vi "Multi_moments_LDA+_An.vi"(3 "Timescales":dbl[](array[numeric]), 4 "Measurement top level?":bool, 6 "Vari Spaced":dbl[][](array[numeric]) format="%.2f") -> (1 "Channel Values":string[](array[string]))   [LabVIEW 2011]
uses:
  Controls/Post_Process.ctl
  Globals/Meas_global.vi
  Globals/Trav_pos_global.vi
  Globals/Dynamic_call_global.ph.vi
  Globals/LDA_meas_global_1.vi
  Acquisition/PWA/PWAtasksGLOBAL.vi
panel:
  out "Channel Names":string[](array[string])
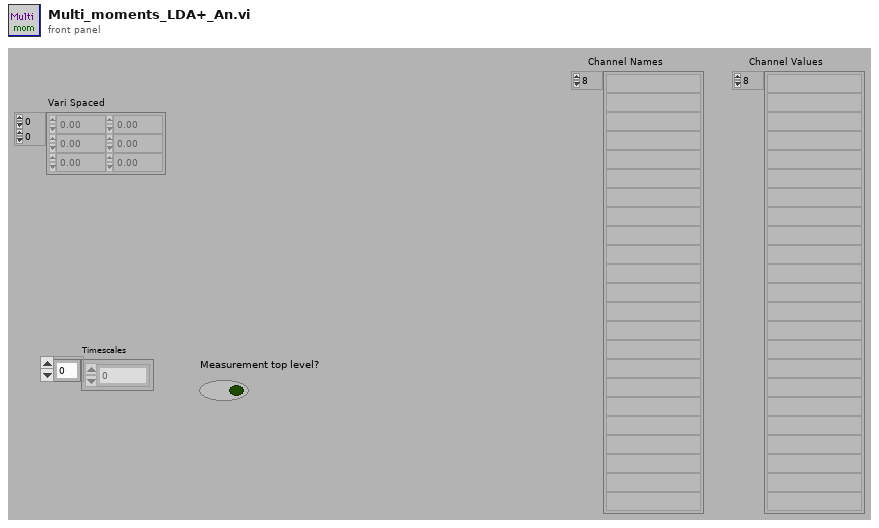
[diagram p1: front panel]
types:
  T1 = typedef "Analysis_info_cluster.ctl" = cluster{"Colour":u32, "Inst type":T2, "Inst name":string, "Symbol":string, "Code name":string, "Extra Info":string, "Inst Array":T3, "Index":i32, "Voltage Index":i32, "Extra Titles":string[], "Extra Values":string[], "Eng Values":dbl[], "Time (ms)":dbl[], "TT / Voltage":dbl[], "U":dbl, "u^2":dbl, "u^3":dbl, "u^4":dbl, "Skew_u":dbl, "Kurt_u":dbl, "Sd Error in Mean":dbl, "% u'/U":dbl, "X":dbl, "Y":dbl, "Z":dbl, "Spectra":T4, "Autocorrelation":T4, "Timescale integral to 25%":dbl, "Sd Error in Variance":dbl, "Calib File":path, "Calib Constants":dbl[], "Histogram":T4, "Output Position":bool, "Full Stats":bool}
  T2 = typedef "Inst_type.ctl" = enum16{"Propeller anemometer", "Raw voltage", "Pressure Transducer", "Pitot-static tube", "Preston tube", "Hot wire", "Cross wire 1", "Cross wire 2", "Generic Linear", "Generic Polynomial", "Generic BackPoly", "Fast FID", "Thermocouple", "Cold wire", "Pulsed Wire", "LDA Vel", "LDA Tran time", "LDA Arr time"}
  T3 = typedef "Instrument_Array.ctl" = enum16{"PWA", "LDA", "Analogue"}
  T4 = typedef "XY_Plot_Cluster.ctl" = cluster{"First Name":string, "Second Name":string, "X axis name":string, "Y axis name":string, "X array":dbl[], "Y array":dbl[]}
  T5 = typedef "Post_Process.ctl" = enum16{"Take New Data", "Post Process Raw Data File"}
  T6 = typedef "PWA_Data.ctl" = enum16{"No PWA Data", "One Ch PWA"}
  T7 = cluster{"Name":string, "X":dbl, "Y":dbl, "Z":dbl}[]
  T8 = typedef "Correlation_cluster1.ctl" = cluster{"U inst":string, "uw":dbl, "u^2w":dbl, "uw^2":dbl, "uw/u'w'":dbl, "W inst":string, "uw^3":dbl, "u^3w":dbl, "u^2w^2":dbl, "Index U":i32, "Index W":i32}
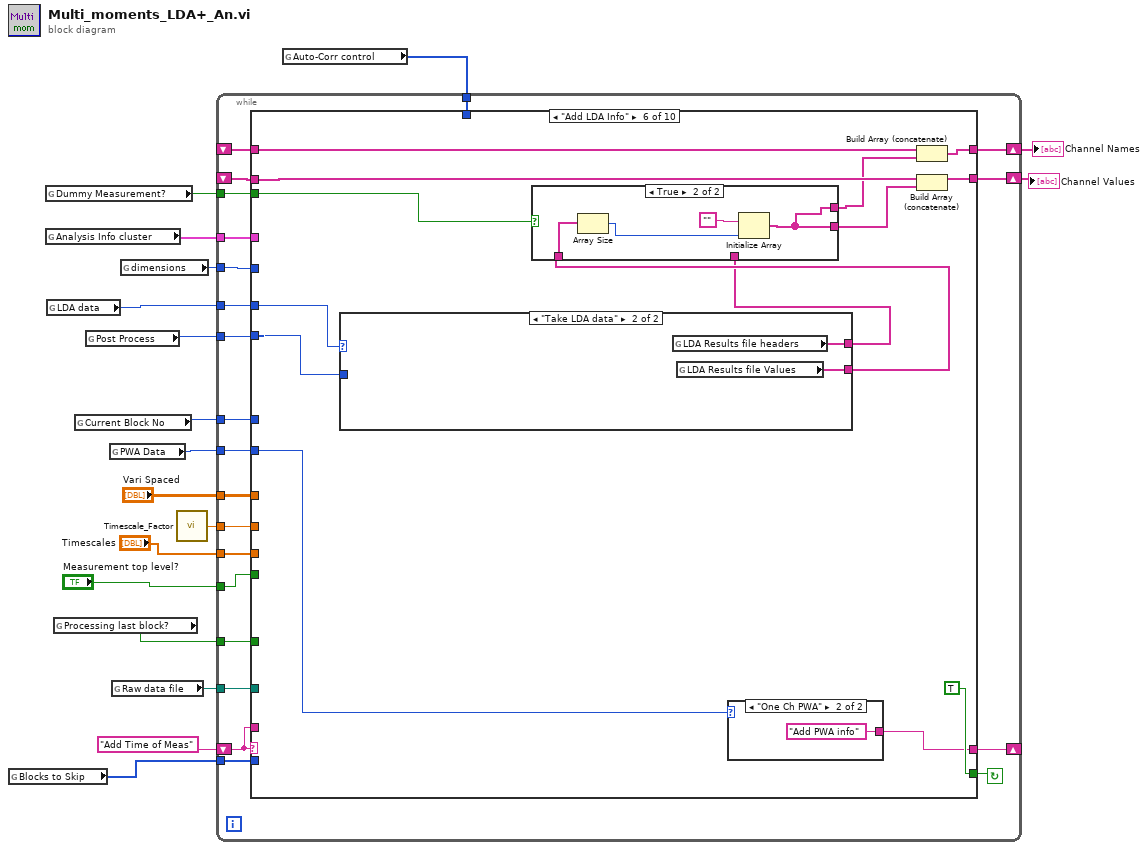
[diagram p0: block diagram]
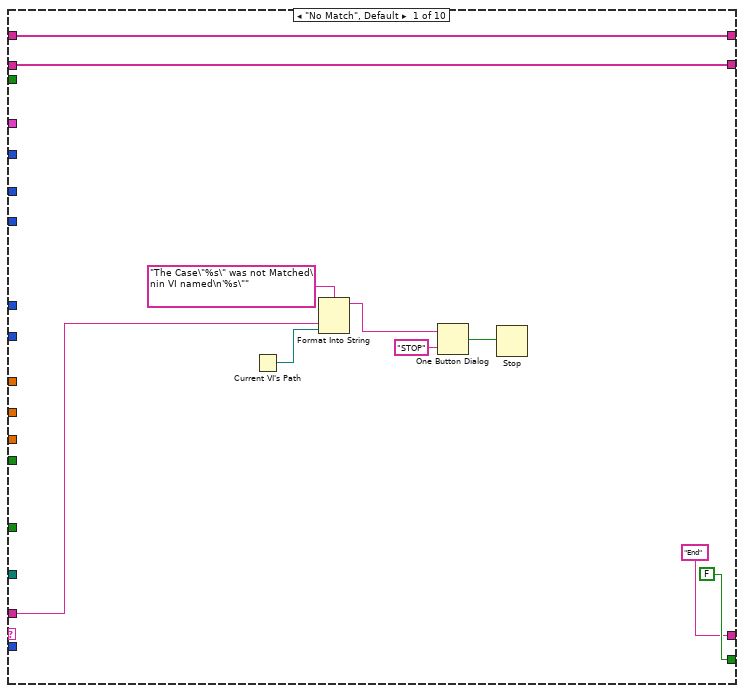
[diagram p2: hidden frame]
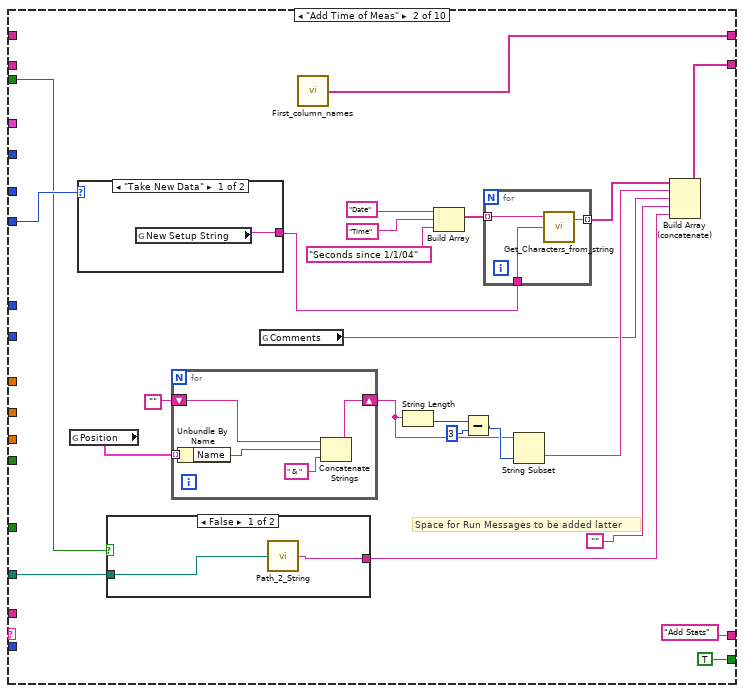
[diagram p3: hidden frame]
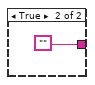
[diagram p4: hidden frame]
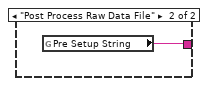
[diagram p5: hidden frame]
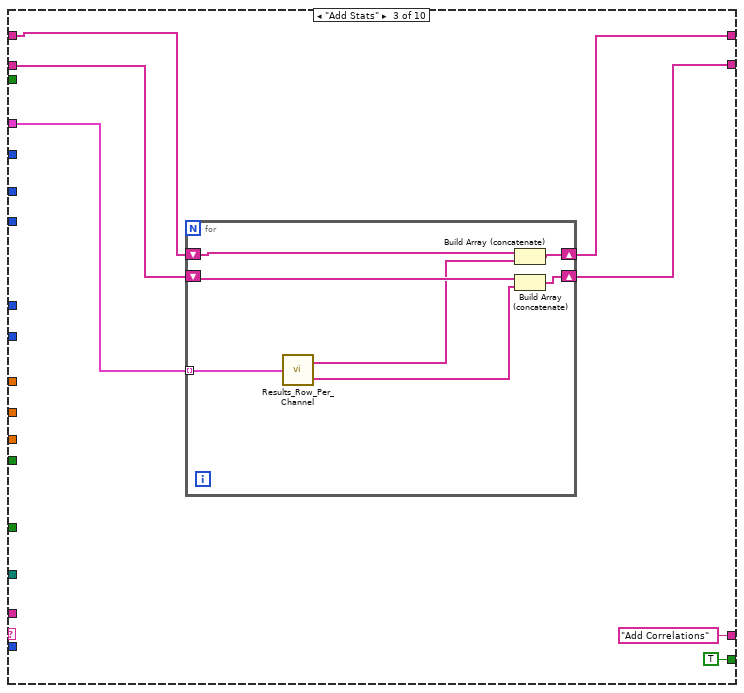
[diagram p6: hidden frame]
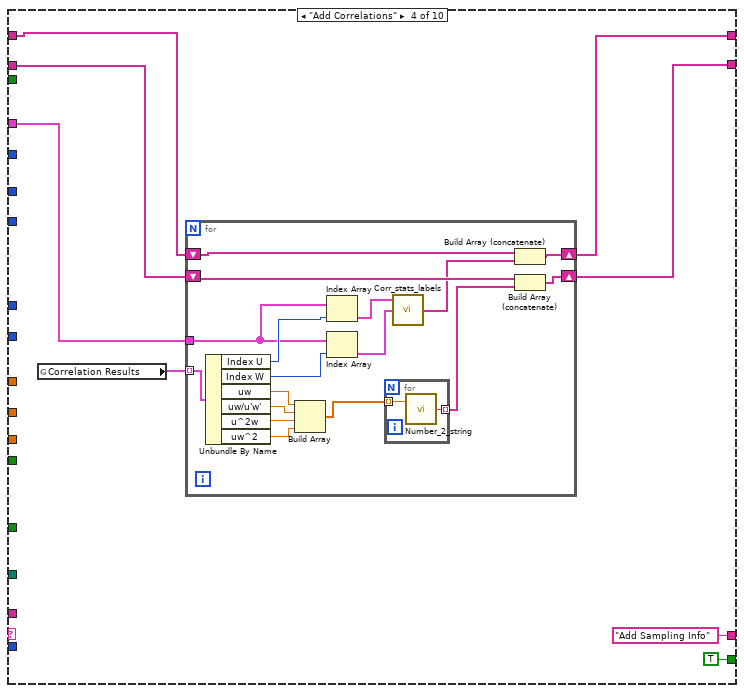
[diagram p7: hidden frame]
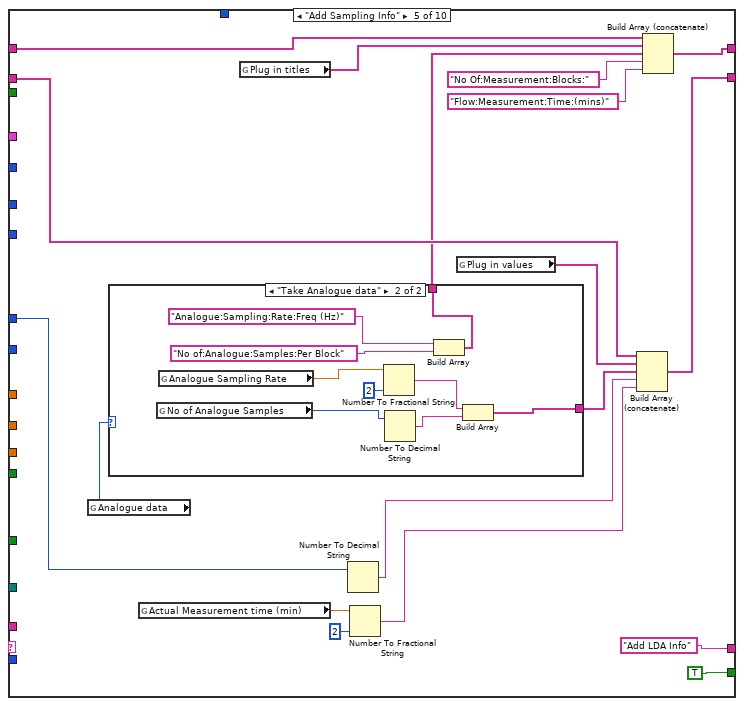
[diagram p8: hidden frame]
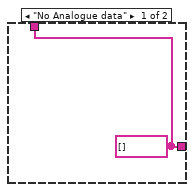
[diagram p9: hidden frame]
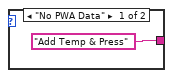
[diagram p10: hidden frame]
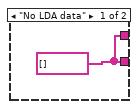
[diagram p12: hidden frame]
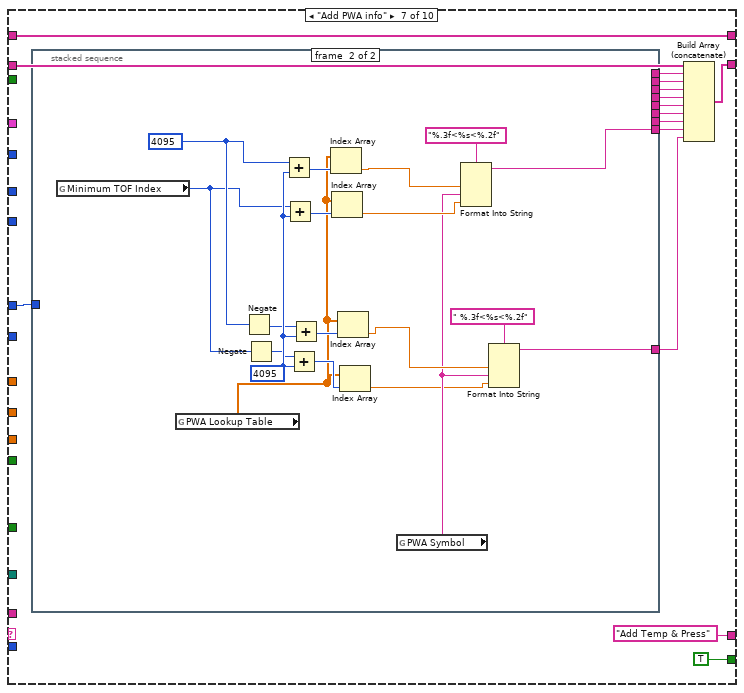
[diagram p13: hidden frame]
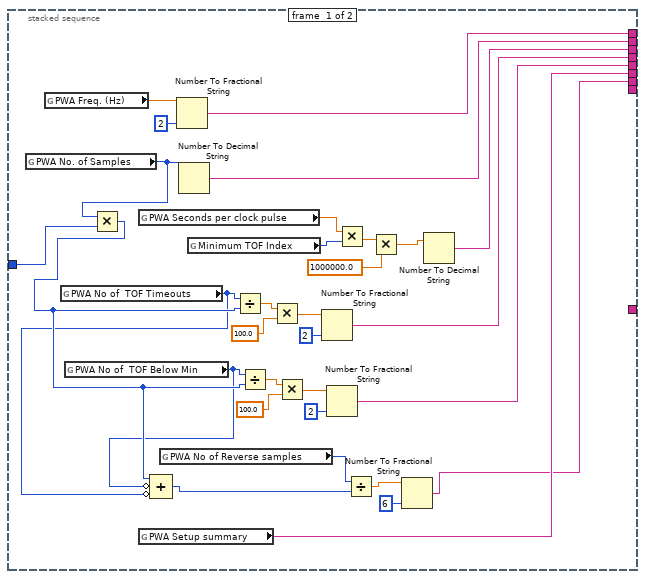
[diagram p14: hidden frame]
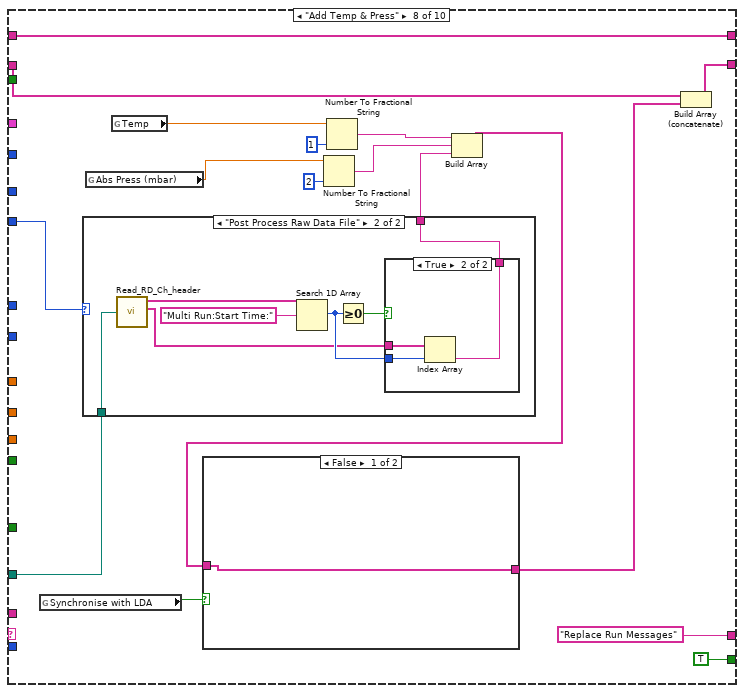
[diagram p15: hidden frame]
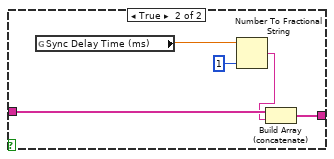
[diagram p16: hidden frame]
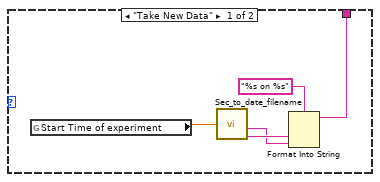
[diagram p17: hidden frame]
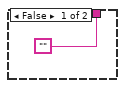
[diagram p18: hidden frame]
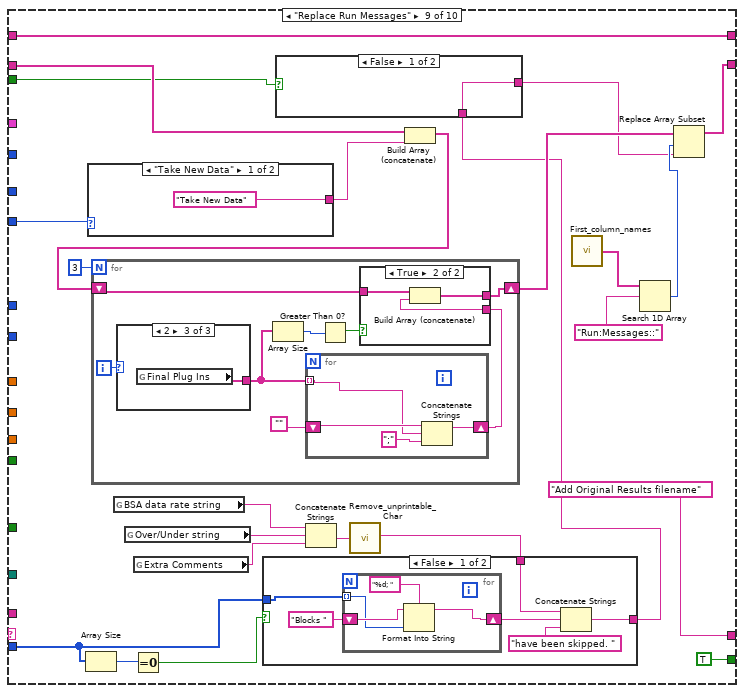
[diagram p19: hidden frame]
diagram:
  n1 = global read "Meas_global.vi" "Blocks to Skip"() -> (w4:i32[])
  n2 = global read "Trav_pos_global.vi" "Dummy Measurement?"() -> (w10:bool)
  n3 = global read "Meas_global.vi" "Analysis Info cluster"() -> (w16:T1[])
  n4 = global read "Meas_global.vi" "LDA data"() -> (w18:enum16{"No LDA data", "Take LDA data"})
  n5 = global read "Meas_global.vi" "Processing last block?"() -> (w12:bool)
  n6 = global read "Meas_global.vi" "Current Block No"() -> (w17:i32)
  n7 = global read "Meas_global.vi" "Post Process"() -> (w15:T5)
  n8 = global read "Meas_global.vi" "PWA Data"() -> (w3:T6)
  n9 = global read "Meas_global.vi" "Raw data file"() -> (w2:path)
  n10 = global read "Meas_global.vi" "dimensions"() -> (w13:enum16{"1D", "2D"})
  n11 = call "Timescale_Factor.vi"() -> ("Factor to scale timescale by"=w5:dbl)
  n12 = global read "Meas_global.vi" "Auto-Corr control"() -> (w7:i32[])
  n13 = while {
    tunnel: "Vari Spaced" -> [w30]
    tunnel: w12 -> [w31]
    tunnel: w13 -> [w32]
    shift-left: _ -> [w33]
    shift-right: [w34] -> w14
    shift-left: "Add Time of Meas" -> [w22]
    shift-right: [w35] -> _
    tunnel: w15 -> [w37]
    tunnel: w16 -> [w38]
    tunnel: w17 -> [w39]
    tunnel: w18 -> [w40]
    tunnel: w10 -> [w29]
    tunnel: "Timescales" -> [w28]
    tunnel: w7 -> [w27]
    shift-right: [w26] -> w1
    shift-left: _ -> [w25]
    tunnel: "Measurement top level?" -> [w24]
    tunnel: w5 -> [w23]
    tunnel: w4 -> [w21]
    tunnel: w3 -> [w20]
    tunnel: w2 -> [w19]
    stop <- w36 continue-if-true
    n14 = case shown="\"Add LDA Info\"" w22 {
      tunnel: w38 -> [_ _ w89 w101 _ _ _ _ _ _]
      tunnel: w40 -> [_ _ _ _ _ w167 _ _ _ _]
      tunnel: w39 -> [_ _ _ _ w139 _ w188 _ _ _]
      tunnel: w37 -> [_ w55 _ _ _ w162 _ w252 w301 w351]
      tunnel: [FALSE ("Processing last block?") TRUE TRUE ("Processing last block?") TRUE ("Processing last block?") TRUE TRUE ("Processing last block?") TRUE ("Processing last block?") TRUE ("Processing last block?") TRUE ("Processing last block?") FALSE] -> w36
      tunnel: ["End" "Add Stats" "Add Correlations" ("t") "Add Sampling Info" ("t") "Add LDA Info" w156 "Add Temp & Press" "Replace Run Messages" "Add Original Results filename" "End"] -> w35
      tunnel: [w42 w72 w90 w105 w138 w168 w191 w261 w304 w348] -> w34
      tunnel: w33 -> [w42 _ w91 w106 w134 w169 w192 w262 w302 w346]
      tunnel: w32 -> [_ _ _ _ _ _ _ _ _ _]
      tunnel: w31 -> [_ _ _ _ _ _ _ _ _ _]
      tunnel: w30 -> [_ _ _ _ _ _ _ _ _ _]
      tunnel: w22 -> [w45 _ _ _ _ _ _ _ _ _]
      tunnel: w29 -> [_ w54 _ _ _ w166 _ _ w292 _]
      tunnel: w28 -> [_ _ _ _ _ _ _ _ _ _]
      tunnel: w27 -> [_ _ _ _ _ _ _ _ _ _]
      tunnel: [w41 w51 w92 w107 w132 w159 w194 w254 w290 w343] -> w26
      tunnel: w25 -> [w41 _ w93 w108 w133 w160 w194 w254 w290 w343]
      tunnel: w24 -> [_ _ _ _ _ _ _ _ _ _]
      tunnel: w23 -> [_ _ _ _ _ _ _ _ _ _]
      tunnel: w21 -> [_ _ _ _ _ _ _ _ w286 _]
      tunnel: w20 -> [_ _ _ _ _ w157 _ _ _ _]
      tunnel: w19 -> [_ w52 _ _ _ _ _ w251 _ _]
      frame "No Match", Default {
        n15 = Current VI's Path() -> (path=w46:path)
        n16 = Format Into String(format string="The Case\"%s\" was not Matched\nin VI named\n'%s\"" ("Format String"), w45, w46) -> (resulting string=w49:string)  [unwired: 2 in, 1 out]
        n17 = One Button Dialog(message=w49, button name ("OK")="STOP") -> (true=w47:bool)
        n18 = Stop(stop? (T)=w47) -> ()
      }
      frame "Add Time of Meas" {
        # "Space for Run Messages to be added latter"
        n19 = global read "Meas_global.vi" "Position"() -> (w62:T7)
        n20 = case shown="\"Take New Data\"" w55 {
          tunnel: [w85 w86] -> w66
          frame "Take New Data" {
            n21 = global read "Meas_global.vi" "New Setup String"() -> (w85:string)
          }
          frame "Post Process Raw Data File" {
            n22 = global read "Meas_global.vi" "Pre Setup String"() -> (w86:string)
          }
        }
        n23 = case shown="False" w54 {
          tunnel: [w75 ""] -> w64
          tunnel: w52 -> [w74 _]
          frame False {
            n24 = call "Path_2_String.vi"("Real Path"=w74) -> ("Path String"=w75:string)
          }
          frame True {
          }
        }
        n25 = for {
          shift-right: [w80] -> w58
          shift-left: "" -> [w81]
          tunnel: w62 -> [w78] mode=indexing
          n26 = Unbundle By Name(w78) -> ("Name"=w77:string)
          n27 = Concatenate Strings(w81, w77, " & ") -> (w80:string)
        }
        n28 = global read "Meas_global.vi" "Comments"() -> (w53:string)
        n29 = call "First_column_names.vi"() -> ("Array"=w51:string[])
        n30 = String Length(string=w58) -> (length=w61:i32)
        n31 = Build Array("Date", "Time", "Seconds since 1/1/04") -> (w68:string[])
        n32 = Subtract(x=w61, y=3) -> (x-y=w59:i32)
        n33 = for {
          tunnel: w68 -> [w84] mode=indexing
          tunnel: w66 -> [w83]
          tunnel: [w82] -> w67 mode=indexing
          n34 = call "Get_Characters_from_string.vi"("Input string"=w83, "Variable name"=w84) -> ("Value"=w82:string)  [unwired: 1 in, 1 out]
        }
        n35 = String Subset(string=w58, length (rest)=w59) -> (substring=w56:string)  [unwired: 1 out]
        n36 = Build Array (concatenate)(w67, w56, w53, "", w64) -> (w72:string[])
      }
      frame "Add Stats" {
        n37 = for {
          shift-right: [w96] -> w92
          shift-left: w93 -> [w99]
          shift-right: [w100] -> w90
          shift-left: w91 -> [w98]
          tunnel: w89 -> [w95] mode=indexing
          n38 = call "Results_Row_Per_Channel.vi"("Analysis_info_cluster"=w95) -> ("Channel Names"=w94:string[], "Channel Values"=w97:string[])
          n39 = Build Array (concatenate)(w99, w94) -> (w96:string[])
          n40 = Build Array (concatenate)(w98, w97) -> (w100:string[])
        }
      }
      frame "Add Correlations" {
        n41 = global read "Meas_global.vi" "Correlation Results"() -> (w102:T8[])
        n42 = for {
          shift-right: [w122] -> w107
          shift-left: w108 -> [w124]
          shift-right: [w125] -> w105
          shift-left: w106 -> [w123]
          tunnel: w102 -> [w121] mode=indexing
          tunnel: w101 -> [w118]
          n43 = Unbundle By Name(w121) -> ("Index U"=w120:i32, "Index W"=w119:i32, "uw"=w114:dbl, "uw/u'w'"=w113:dbl, "u^2w"=w112:dbl, "uw^2"=w111:dbl)
          n44 = Build Array(w114, w113, w112, w111) -> (w110:dbl[])
          n45 = Index Array(array=w118, index=w120) -> (element=w117:T1)
          n46 = Index Array(array=w118, index=w119) -> (element=w116:T1)
          n47 = for {
            tunnel: w110 -> [w127] mode=indexing
            tunnel: [w126] -> w109 mode=indexing
            n48 = call "Number_2_string.vi"("number"=w127) -> ("String"=w126:string)  [unwired: 1 in]
          }
          n49 = call "Corr_stats_labels.vi"("Inst 2 Units"=w116, "Inst 1 Units"=w117) -> ("Output"=w115:string[])  [unwired: 1 in]
          n50 = Build Array (concatenate)(w124, w115) -> (w122:string[])
          n51 = Build Array (concatenate)(w123, w109) -> (w125:string[])
        }
      }
      frame "Add Sampling Info" {
        n52 = global read "Meas_global.vi" "Analogue data"() -> (w143:enum16{"No Analogue data", "Take Analogue data"})
        n53 = case shown="\"Take Analogue data\"" w143 {
          tunnel: [w146 w150] -> w136
          tunnel: [w146 w147] -> w130
          frame "No Analogue data" {
            w146 = string[] []
          }
          frame "Take Analogue data" {
            n54 = global read "Meas_global.vi" "No of Analogue Samples"() -> (w153:i32)
            n55 = global read "Meas_global.vi" "Analogue Sampling Rate"() -> (w154:dbl)
            n56 = Number To Fractional String(number=w154, precision (6)=i16 2) -> (F-format string=w152:string)  [unwired: 2 out]
            n57 = Number To Decimal String(number=w153) -> (decimal integer string=w151:string)  [unwired: 1 out]
            n58 = Build Array("Analogue:Sampling:Rate:Freq (Hz)", "No of:Analogue:Samples:Per Block") -> (w147:string[])
            n59 = Build Array(w152, w151) -> (w150:string[])
          }
        }
        n60 = global read "Meas_global.vi" "Actual Measurement time (min)"() -> (w140:dbl)
        n61 = global read "Dynamic_call_global.ph.vi" "Plug in titles"() -> (w131:string[])
        n62 = Number To Decimal String(number=w139) -> (decimal integer string=w137:string)  [unwired: 1 out]
        n63 = Number To Fractional String(number=w140, precision (6)=i16 2) -> (F-format string=w142:string)  [unwired: 2 out]
        n64 = global read "Dynamic_call_global.ph.vi" "Plug in values"() -> (w135:string[])
        n65 = Build Array (concatenate)(w134, w135, w136, w137, w142) -> (w138:string[])
        n66 = Build Array (concatenate)(w133, w131, w130, "No Of:Measurement:Blocks:", "Flow:Measurement:Time:(mins)") -> (w132:string[])
      }
      frame "Add LDA Info" {
        n67 = case shown="\"Take LDA data\"" w167 {
          tunnel: w162 -> [_ _]
          tunnel: [w178 w180] -> w163
          tunnel: [w178 w179] -> w161
          frame "No LDA data" {
            w178 = string[] []
          }
          frame "Take LDA data" {
            n68 = global read "LDA_meas_global_1.vi" "LDA Results file headers"() -> (w179:string[])
            n69 = global read "LDA_meas_global_1.vi" "LDA Results file Values"() -> (w180:string[])
          }
        }
        n70 = case shown="True" w166 {
          tunnel: [w173 w174] -> w165
          tunnel: w163 -> [w173 w177]
          tunnel: [w172 w174] -> w158
          tunnel: w161 -> [w172 _]
          frame False {
          }
          frame True {
            n71 = Array Size(array=w177) -> (size(s)=w176:i32)
            n72 = Initialize Array("", w176) -> (w174:string[])
          }
        }
        n73 = case shown="\"One Ch PWA\"" w157 {
          tunnel: ["Add Temp & Press" "Add PWA info"] -> w156
          frame "No PWA Data" {
          }
          frame "One Ch PWA" {
          }
        }
        n74 = Build Array (concatenate)(w160, w158) -> (w159:string[])
        n75 = Build Array (concatenate)(w169, w165) -> (w168:string[])
      }
      frame "Add PWA info" {
        n76 = stacked-sequence {
          tunnel: [w225 _] -> w190
          tunnel: [w223 _] -> w189
          tunnel: w188 -> [w221 _]
          tunnel: [w216 _] -> w187
          tunnel: [w211 _] -> w186
          tunnel: [w210 _] -> w185
          tunnel: [_ w228] -> w184
          tunnel: [_ w227] -> w183
          tunnel: [w204 _] -> w182
          tunnel: [w196 _] -> w181
          frame #0 {
            n77 = global read "PWAtasksGLOBAL.vi" "PWA No. of Samples"() -> (w222:i32)
            n78 = global read "PWAtasksGLOBAL.vi" "PWA Freq. (Hz)"() -> (w226:dbl)
            n79 = global read "PWAtasksGLOBAL.vi" "PWA No of  TOF Timeouts"() -> (w201:i32)
            n80 = global read "PWAtasksGLOBAL.vi" "PWA No of  TOF Below Min"() -> (w202:i32)
            n81 = Multiply(x=w222, y=w221) -> (x*y=w203:i32)
            n82 = global read "PWAtasksGLOBAL.vi" "PWA Seconds per clock pulse"() -> (w208:dbl)
            n83 = global read "PWAtasksGLOBAL.vi" "PWA Setup summary"() -> (w210:string)
            n84 = Compound Arithmetic op=ADD(w203, invert w202, invert w201) -> (w199:i32)
            n85 = global read "PWAtasksGLOBAL.vi" "PWA No of Reverse samples"() -> (w200:i32)
            n86 = Number To Fractional String(number=w226, precision (6)=i16 2) -> (F-format string=w225:string)  [unwired: 2 out]
            n87 = Number To Decimal String(number=w222) -> (decimal integer string=w223:string)  [unwired: 1 out]
            n88 = global read "PWAtasksGLOBAL.vi" "Minimum TOF Index"() -> (w209:i16)
            n89 = Divide(x=w201, y=w203) -> (x/y=w220:dbl)
            n90 = Divide(x=w202, y=w203) -> (x/y=w212:dbl)
            n91 = Multiply(x=w220, y=100.0) -> (x*y=w217:dbl)
            n92 = Multiply(x=w212, y=100.0) -> (x*y=w215:dbl)
            n93 = Number To Fractional String(number=w217, precision (6)=i16 2) -> (F-format string=w216:string)  [unwired: 2 out]
            n94 = Number To Fractional String(number=w215, precision (6)=i16 2) -> (F-format string=w211:string)  [unwired: 2 out]
            n95 = Multiply(x=w208, y=w209) -> (x*y=w207:dbl)
            n96 = Divide(x=w200, y=w199) -> (x/y=w197:dbl)
            n97 = Multiply(x=w207, y=1000000.0) -> (x*y=w205:dbl)
            n98 = Number To Fractional String(number=w197, precision (6)=i16 6) -> (F-format string=w196:string)  [unwired: 2 out]
            n99 = Number To Decimal String(number=w205) -> (decimal integer string=w204:string)  [unwired: 1 out]
          }
          frame #1 {
            w241 = 4095
            w237 = 4095
            n100 = global read "PWAtasksGLOBAL.vi" "Minimum TOF Index"() -> (w236:i16)
            n101 = global read "PWAtasksGLOBAL.vi" "PWA Lookup Table"() -> (w240:dbl[])
            n102 = Negate(x=w237) -> (-x=w239:i32)
            n103 = Negate(x=w236) -> (-x=w238:i16)
            n104 = Add(x=w237, y=w241) -> (x+y=w242:i32)
            n105 = Add(x=w236, y=w241) -> (x+y=w243:i32)
            n106 = Add(x=w238, y=w241) -> (x+y=w245:i32)
            n107 = Add(x=w239, y=w241) -> (x+y=w244:i32)
            n108 = Index Array(array=w240, index=w242) -> (element=w235:dbl)
            n109 = Index Array(array=w240, index=w243) -> (element=w234:dbl)
            n110 = Index Array(array=w240, index=w244) -> (element=w231:dbl)
            n111 = Index Array(array=w240, index=w245) -> (element=w229:dbl)
            n112 = global read "PWAtasksGLOBAL.vi" "PWA Symbol"() -> (w230:string)
            n113 = Format Into String(format string="%.3f<%s<%.2f", w235, w230, w234) -> (resulting string=w228:string)  [unwired: 2 in, 1 out]
            n114 = Format Into String(format string=" %.3f<%s<%.2f", w231, w230, w229) -> (resulting string=w227:string)  [unwired: 2 in, 1 out]
          }
        }
        n115 = Build Array (concatenate)(w192, w190, w189, w182, w187, w186, w185, w181, w184, w183) -> (w191:string[])
      }
      frame "Add Temp & Press" {
        n116 = global read "Meas_global.vi" "Synchronise with LDA"() -> (w249:bool)
        n117 = case shown="\"Post Process Raw Data File\"" w252 {
          tunnel: [w269 w274] -> w253
          tunnel: w251 -> [_ w280]
          frame "Take New Data" {
            n118 = global read "Meas_global.vi" "Start Time of experiment"() -> (w273:dbl)
            n119 = call "Sec_to_date_filename.vi"("seconds"=w273) -> ("Day"=w271:string, "Time"=w272:string)  [unwired: 2 out]
            n120 = Format Into String(format string="%s on %s", w272, w271) -> (resulting string=w269:string)  [unwired: 2 in, 1 out]
          }
          frame "Post Process Raw Data File" {
            n121 = call "Read_RD_Ch_header.vi"("Raw data file"=w280) -> ("Ch Name Out"=w279:string[], "Ch Values"=w275:string[])  [unwired: 2 out]
            n122 = Search 1D Array(1D array=w279, element="Multi Run:Start Time:") -> (index of element=w276:i32)  [unwired: 1 out]
            n123 = Greater Or Equal To 0?(x=w276) -> (x >= 0?=w277:bool)
            n124 = case shown="True" w277 {
              tunnel: w276 -> [_ w284]
              tunnel: w275 -> [_ w283]
              tunnel: ["" w282] -> w274
              frame False {
              }
              frame True {
                n125 = Index Array(array=w283, index=w284) -> (element=w282:string)
              }
            }
          }
        }
        n126 = global read "Meas_global.vi" "Abs Press (mbar)"() -> (w259:dbl)
        n127 = global read "Meas_global.vi" "Temp"() -> (w255:dbl)
        n128 = Number To Fractional String(number=w259, precision (6)=i16 2) -> (F-format string=w260:string)  [unwired: 2 out]
        n129 = Number To Fractional String(number=w255, precision (6)=i16 1) -> (F-format string=w257:string)  [unwired: 2 out]
        n130 = Build Array(w257, w260, w253) -> (w247:string[])
        n131 = case shown="False" w249 {
          tunnel: w247 -> [w263 w266]
          tunnel: [w263 w264] -> w246
          frame False {
          }
          frame True {
            n132 = global read "LDA_meas_global_1.vi" "Sync Delay Time (ms)"() -> (w267:dbl)
            n133 = Number To Fractional String(number=w267, precision (6)=i16 1) -> (F-format string=w265:string)  [unwired: 2 out]
            n134 = Build Array (concatenate)(w266, w265) -> (w264:string[])
          }
        }
        n135 = Build Array (concatenate)(w262, w246) -> (w261:string[])
      }
      frame "Replace Run Messages" {
        n136 = Array Size(array=w286) -> (size(s)=w287:i32)
        n137 = case shown="\"Take New Data\"" w301 {
          tunnel: ["Take New Data" "Post Process"] -> w300
          frame "Take New Data" {
          }
          frame "Post Process Raw Data File" {
          }
        }
        n138 = global read "Meas_global.vi" "BSA data rate string"() -> (w306:string)
        n139 = global read "Meas_global.vi" "Over/Under string"() -> (w308:string)
        n140 = Equal To 0?(x=w287) -> (x = 0?=w285:bool)
        n141 = global read "Meas_global.vi" "Extra Comments"() -> (w307:string)
        n142 = Concatenate Strings(w306, w308, w307) -> (w305:string)
        n143 = call "Remove_unprintable_Char.vi"("Input String"=w305) -> ("Output String"=w289:string)
        n144 = case shown="False" w285 {
          tunnel: w286 -> [w314 _]
          tunnel: w289 -> [w310 w319]
          tunnel: [w309 w319] -> w288
          frame False {
            n145 = for {
              shift-right: [w316] -> w312
              shift-left: "Blocks " -> [w318]
              tunnel: w314 -> [w317] mode=indexing
              n146 = Format Into String(format string="%d; ", initial string=w318, w317) -> (resulting string=w316:string)  [unwired: 1 in, 1 out]
            }
            n147 = Concatenate Strings(w310, w312, "have been skipped. " ("string")) -> (w309:string)
          }
          frame True {
          }
        }
        n148 = case shown="False" w292 {
          tunnel: [w320 "Dummy Measurement"] -> w291
          tunnel: w288 -> [w320 _]
          frame False {
          }
          frame True {
          }
        }
        n149 = Build Array (concatenate)(w302, w300) -> (w297:string[])
        n150 = for {
          N: 3 -> [_]
          shift-right: [w324] -> w296
          shift-left: w297 -> [w325]
          i -> [w328]
          n151 = case shown="2" w328 {
            tunnel: [w334 w335 w336] -> w322
            frame 0, Default {
              n152 = global read "Dynamic_call_global.ph.vi" "Initial Plug Ins"() -> (w334:string[])
            }
            frame 1 {
              n153 = global read "Dynamic_call_global.ph.vi" "Per Block Plug Ins"() -> (w335:string[])
            }
            frame 2 {
              n154 = global read "Dynamic_call_global.ph.vi" "Final Plug Ins"() -> (w336:string[])
            }
          }
          n155 = Array Size(array=w322) -> (size(s)=w327:i32)
          n156 = for {
            tunnel: w322 -> [w337] mode=indexing
            shift-right: [w338] -> w323
            shift-left: "" -> [w340]
            n157 = Concatenate Strings(w340, w337, ";" ("string")) -> (w338:string)
          }
          n158 = Greater Than 0?(x=w327) -> (x > 0?=w326:bool)
          n159 = case shown="True" w326 {
            tunnel: w325 -> [w330 w333]
            tunnel: [w330 w332] -> w324
            tunnel: w323 -> [_ w331]
            frame False {
            }
            frame True {
              n160 = Build Array (concatenate)(w333, w331) -> (w332:string[])
            }
          }
        }
        n161 = call "First_column_names.vi"() -> ("Array"=w295:string[])
        n162 = Search 1D Array(1D array=w295, element="Run:Messages::") -> (index of element=w294:i32)  [unwired: 1 out]
        n163 = Replace Array Subset(array=w296, new element=w291, index=w294) -> (w304:string[])
      }
      frame "Add Original Results filename" {
        n164 = Equal?(x=w351, y=Post_Process."Take New Data" ("Post Process")) -> (x = y?=w350:bool)
        n165 = case shown="False" w350 {
          tunnel: [w353 w357] -> w345
          frame False {
            n166 = global read "Meas_global.vi" "Pre Setup String"() -> (w356:string)
            n167 = call "Get_Characters_from_string.vi"("Input string"=w356, "Variable name"="Results filename") -> ("Value"=w354:string)  [unwired: 1 in, 1 out]
            n168 = call "String_to_Pathname.vi"("Input String"=w354) -> ("path"=w353:path)
          }
          frame True {
            n169 = global read "Meas_global.vi" "Results file"() -> (w357:path)
          }
        }
        n170 = Strip Path(path=w345) -> (name=w344:string)  [unwired: 1 out]
        n171 = Build Array (concatenate)(w346, w344) -> (w348:string[])
      }
    }
  }
  "Channel Values" <- w14
  "Channel Names" <- w1
